vi "(SubVI) Acquire Sinewave True Amplitude A by using Waveform WriteRead_PI_YCC.vi"(5 "f_drive (Hz)":dbl=32.0, 6 "Amplitude, A (nm)":dbl=500.0, 7 "Axis  (Enum)":enum16{"x", "y", "z"}(ring)) -> (1 "True f_drive (Hz)":dbl, 2 "True Amplitude, A (nm)":dbl)   [LabVIEW 2014]
uses:
  <vilib>/Utility/file.llb/Write To Spreadsheet File (DBL).vi
panel:
  out "Cut-Position Array (um)":dbl[](array[numeric])
  out "Cut-Time Array (s)":dbl[](array[numeric])
  out "Start Position (um)":dbl format="%0.5f"
  in  "Tab Control":enum32{"Command", "True Output", "Fitting"}(tab)
  out "Commanded XY Graph":cluster{dbl[], "Data Array Out to read":dbl[]}(graph)
  out "Read XY Graph":cluster{dbl[], "Data Array Out to read":dbl[]}(graph)
  out "Read XY Graph 2":cluster{dbl[], "Data Array Out to read":dbl[]}[](graph)
  out "best nonlinear fit for cut position":dbl[](array[numeric])
  in  "Save?":bool
  out "Read Position Array (um)":dbl[](array[numeric])
  out "Time Array (s)":dbl[](array[numeric])
  out "Sampling Rate (Hz)":dbl
  out "best fit parameters":dbl[](array[numeric])
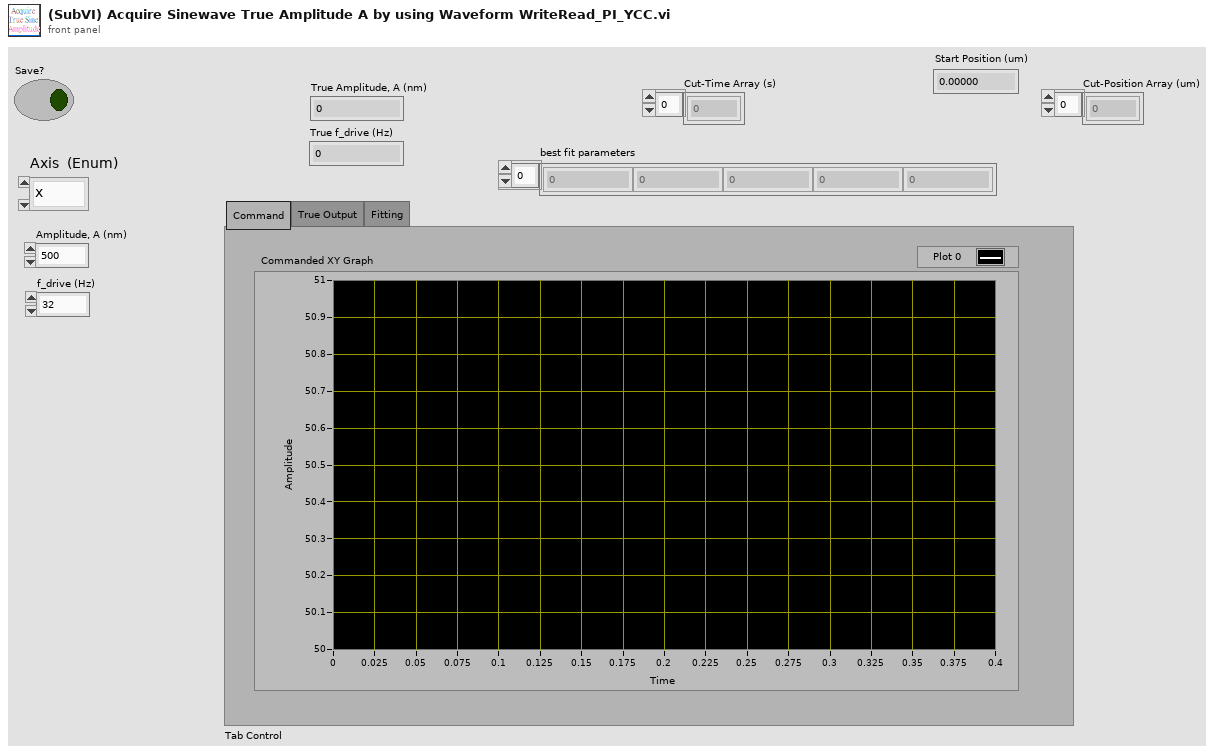
[diagram p1: front panel]
types:
  T1 = cluster{"Time Array (s)":dbl[], "Target Positions Array (um)":dbl[]}
  T2 = cluster{"Time Array (s)":dbl[], "Read Positions Array (um)":dbl[]}
  T3 = cluster{"Cut-Time Array (s)":dbl[], "Cut-Position Array (um)":dbl[]}
  T4 = cluster{"Cut-Time Array (s)":dbl[], "best nonlinear fit for cut position":dbl[]}
  T5 = cluster{"Cut-Time Array (s)":dbl[], "best nonlinear fit for cut position":dbl[]}[]
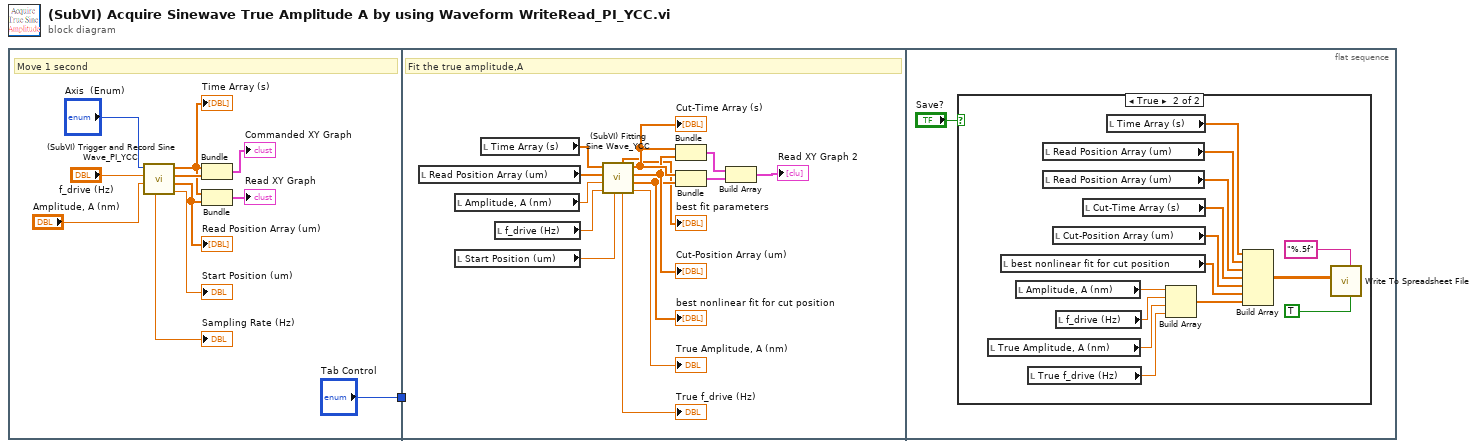
[diagram p0: block diagram]
diagram:
  n1 = flat-sequence {
    tunnel: ["Tab Control"] -> w1
    tunnel: w1 -> [_]
    frame #0 {
      # "Move 1 second"
      # "Cut 1/3~2/3 data to fit"
      n2 = call "(SubVI) Trigger and Record Sine Wave_PI_YCC.vi"("Amplitude (nm)"="Amplitude, A (nm)", "freq. (Hz)"="f_drive (Hz)", "Axis  (Enum)"="Axis  (Enum)") -> ("Start Position (um)"=→"Start Position (um)":dbl, "Read Positions Array (um)"=w3:dbl[], "Target Positions Array (um)"=w8:dbl[], "Time Array (s)"=w4:dbl[], "DAC rate (Hz)"=→"Sampling Rate (Hz)":dbl)  [unwired: 2 in]
      "Time Array (s)" <- w4
      "Read Position Array (um)" <- w3
      n3 = Bundle("Time Array (s)"=w4, "Target Positions Array (um)"=w8) -> (→"Commanded XY Graph":T1)  [unwired: 1 in]
      n4 = Bundle("Time Array (s)"=w4, "Read Positions Array (um)"=w3) -> (→"Read XY Graph":T2)  [unwired: 1 in]
    }
    frame #1 {
      # "Fit the true amplitude,A"
      n5 = local read "Read Position Array (um)"() -> (w19:dbl[])
      n6 = local read "Amplitude, A (nm)"() -> (w22:dbl)
      n7 = local read "Start Position (um)"() -> (w24:dbl)
      n8 = local read "Time Array (s)"() -> (w20:dbl[])
      n9 = local read "f_drive (Hz)"() -> (w23:dbl)
      n10 = call "(SubVI) Fitting Sine Wave_YCC.vi"("Start Position (um)"=w24, "f_drive (Hz)"=w23, "Amplitude, A (nm)"=w22, "Position array (um)"=w19, "Time array (s)"=w20) -> ("True Amplitude, A (nm)"=→"True Amplitude, A (nm)":dbl, "best nonlinear fit for cut position"=w16:dbl[], "Cut-Position Array (um)"=w17:dbl[], "Cut-Time Array (s)"=w18:dbl[], "True f_drive (Hz)"=→"True f_drive (Hz)":dbl, "best fit parameters"=→"best fit parameters":dbl[])  [unwired: 1 in]
      "best nonlinear fit for cut position" <- w16
      "Cut-Time Array (s)" <- w18
      "Cut-Position Array (um)" <- w17
      n11 = Bundle("Cut-Time Array (s)"=w18, "Cut-Position Array (um)"=w17) -> (w21:T3)  [unwired: 1 in]
      n12 = Bundle("Cut-Time Array (s)"=w18, "best nonlinear fit for cut position"=w16) -> (w25:T4)  [unwired: 1 in]
      n13 = Build Array(w21, w25) -> (→"Read XY Graph 2":T5)
    }
    frame #2 {
      n14 = case shown="True" "Save?" {
        frame False {
        }
        frame True {
          n15 = local read "True Amplitude, A (nm)"() -> (w33:dbl)
          n16 = local read "best nonlinear fit for cut position"() -> (w36:dbl[])
          n17 = local read "Amplitude, A (nm)"() -> (w35:dbl)
          n18 = local read "True f_drive (Hz)"() -> (w32:dbl)
          n19 = local read "Read Position Array (um)"() -> (w40:dbl[])
          n20 = local read "Read Position Array (um)"() -> (w39:dbl[])
          n21 = local read "Cut-Position Array (um)"() -> (w37:dbl[])
          n22 = local read "f_drive (Hz)"() -> (w34:dbl)
          n23 = local read "Cut-Time Array (s)"() -> (w38:dbl[])
          n24 = local read "Time Array (s)"() -> (w41:dbl[])
          n25 = Build Array(w35, w34, w33, w32) -> (w31:dbl[])
          n26 = Build Array(w41, w40, w39, w38, w37, w36, w31) -> (w30:dbl[][])
          n27 = call-poly <vilib>:"Write To Spreadsheet File.vi"("transpose? (no:F)"=TRUE, "format (%.3f)"="%.5f", "2D data"=w30) -> ()  [unwired: 5 in, 1 out]
        }
      }
    }
  }
